vi "CalculateDiscountPercentage.vi"(8 "Error In":errorcluster, 10 "Customer":refnum<class "Customer.lvclass">, 11 "reference in":refnum<class "DiscountRuleEngine.lvclass">) -> (0 "Error Out":errorcluster, 2 "Return(EXT)":ext, 3 "reference out":refnum<class "DiscountRuleEngine.lvclass">)   [LabVIEW 2020, in "DiscountRuleEngine.lvclass"]
uses:
  DiscountRuleEngine.lvclass
  Customer_class/Customer.lvclass
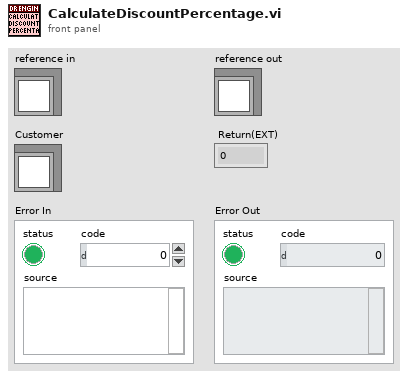
[diagram p1: front panel]
types:
  T1 = typedef "DiscountRuleEngine.lvclass/ObjectAttributes.ctl" = cluster{"_rules":refnum<class "IDiscountRule.lvclass">[], "_priorityRules":refnum<class "IExclusivePriorityRule.lvclass">[]}
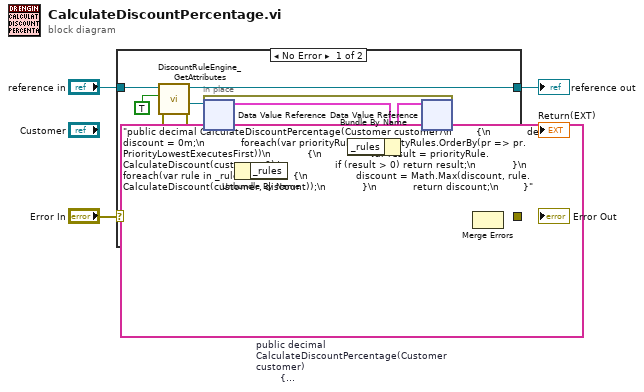
[diagram p0: block diagram]
diagram:
  (unwired) "public decimal CalculateDiscountPercentage(Customer customer)\n        {\n            decimal discount = 0m;\n            foreach(var priorityRule in _priorityRules.OrderBy(pr => pr.PriorityLowestExecutesFirst))\n            {\n                var result = priorityRule.CalculateDiscount(customer, 0);\n                if (result > 0) return result;\n            }\n            foreach(var rule in _rules)\n            {\n                discount = Math.Max(discount, rule.CalculateDiscount(customer, discount));\n            }\n            return discount;\n        }"  # public decimal CalculateDiscountPercentage(Customer customer)         {             decimal discount = 0m;             foreach(var priorityRule in _priorityRules.OrderBy(pr => pr.PriorityLowestExecutesFirst))             {                 var result = priorityRule.CalculateDiscount(customer, 0);                 if (result > 0) return result;             }             foreach(var rule in _rules)             {                 discount = Math.Max(discount, rule.CalculateDiscount(customer, discount));             }             return discount;         }
  n1 = case shown="No Error" "Error In" {
    selector: "Error In" -> [w11 w16]
    tunnel: [w8 w16] -> w3
    tunnel: [w9 w15] -> w1
    tunnel: "reference in" -> [w12 w15]
    frame No Error {
      n2 = call "DiscountRuleEngine_GetAttributes.vi"("error in (no error)"=w11, "OnlyGetDvrReference(False)"=TRUE, "reference in"=w12) -> ("error out"=w6:errorcluster, "DataRef"=w7:refnum<data-value>, "reference out"=w9:refnum<class "DiscountRuleEngine.lvclass">)  [unwired: 5 in, 1 out]
      n3 = in-place {
        n4 = in-place-dvr #1(w7) -> (w13:T1)  [unwired: 1 out]
        n5 = Unbundle By Name(w13) -> ()  [unwired: 1 out]
        n6 = Bundle By Name(cluster=w13) -> (w14:T1)  [unwired: 1 in]
        n7 = in-place-dvr #1(w14) -> (w10:errorcluster)  [unwired: 1 out]
      }
      n8 = Merge Errors(w6, w10) -> (w8:errorcluster)
    }
    frame Error {
    }
  }
  "Error Out" <- w3
  "reference out" <- w1
